vi "KE6221 -- Set Arb Wave Params.vi"(0 "Resource In":refnum<visa-resource-name>, 1 "Check For SCPI Errors? (T)":bool=TRUE, 5 "Arb Location":T1, 7 "Arb Wave Params In":T2={"Frequency (Hz)"=1000.0, "Amplitude (A)"=0.001, "Offset (A)"=0.0, "Ranging Mode"=enum."Best", "Fixed Range"=enum."2mA", "Playback Mode"=enum."Time", "Time (s)"=1.0, "Num Cycles"=1.0, "Phase\nMarker?"=FALSE, "Phase Marker (deg)"=180.0, "Trig Link Line"=enum."1", "Arb Waveform Points"=[], "Num Arb Points"=0} {"Arb Waveform Points" min=-1.0 max=1.0 format="%.3f"; "Offset (A)" min=-0.105 max=0.105 format="%.4p"; "Num Cycles" min=0.001 max=99999999900.0 format="%.3p"; "Time (s)" min=1e-07 max=999999.999 format="%.3p"; "Phase Marker (deg)" min=0.0 max=360.0 format="%.3f"; "Amplitude (A)" min=2e-12 max=0.105 format="%.3p"; "Frequency (Hz)" min=0.001 max=100000.0 format="%.3p"}, 11 "error in (no error)":errorcluster, 12 "Read Back Set Values? (T)":bool=TRUE, 13 "Timeout (10000 ms)":u32=10000) -> (4 "Resource Out (dupl)":refnum<visa-resource-name>, 8 "Arb Wave Params Out":T2={"Frequency (Hz)"=1000.0, "Amplitude (A)"=0.001, "Offset (A)"=0.0, "Ranging Mode"=enum."Best", "Fixed Range"=enum."2mA", "Playback Mode"=enum."Time", "Time (s)"=1.0, "Num Cycles"=1.0, "Phase\nMarker?"=FALSE, "Phase Marker (deg)"=180.0, "Trig Link Line"=enum."1", "Arb Waveform Points"=[], "Num Arb Points"=0} {"Arb Waveform Points" min=-1.0 max=1.0 format="%.3f"; "Offset (A)" min=-0.105 max=0.105 format="%.4p"; "Num Cycles" min=0.001 max=99999999900.0 format="%.3p"; "Time (s)" min=1e-07 max=999999.999 format="%.3p"; "Phase Marker (deg)" min=0.0 max=360.0 format="%.3f"; "Amplitude (A)" min=2e-12 max=0.105 format="%.3p"; "Frequency (Hz)" min=0.001 max=100000.0 format="%.3p"}, 15 "error out":errorcluster)   [LabVIEW 2019, in "Keithley 622x.lvlib"]
doc: "Sets the parameters for an arbitray ('Arb') wave. The user must specify the memory location he wants to write the waveform to, and if it's anything other tha '0 (Volatile)', the waveform will be automatically copied to the non-voltage memory location specified. Note that this VI can only be used with the 6221, since the 6220 doesn't support this feature."
uses:
  Keithley 622x.lvlib
  Typedefs/KE6221 -- Wave Arb Wave Params.ctl
  Low Level/Typedefs/KE6221 -- Wave Frequency.ctl
  Low Level/Typedefs/KE6221 -- Wave Amplitude.ctl
  Source/Typedefs/KE622x -- Current Level.ctl
  Low Level/Typedefs/KE6221 -- Wave Ranging Mode.ctl
  Source/Typedefs/KE622x -- Current Ranges.ctl
  Low Level/Typedefs/KE6221 -- Wave Playback Mode.ctl
  Low Level/Typedefs/KE6221 -- Wave Playback Time.ctl
  Low Level/Typedefs/KE6221 -- Wave Playback Num Cycles.ctl
  Low Level/Typedefs/KE6221 -- Wave Phase Marker.ctl
  Trigger/Low Level/Typedefs/KE622x -- Trig Link Line.ctl
  Low Level/Typedefs/KE6221 -- Wave Arb Point.ctl
  Low Level/Typedefs/KE6221 -- Arb Location.ctl
  Low Level/Typedefs/KE6221 -- Wave Type.ctl
  Source/Typedefs/KE622x -- Current Range.ctl
panel:
  # "Note:  \"Arb Waveform Points\" and \"Num Arb Points\" refer to the Arb waveform in volatile memory (a.k.a. 'Location 0'). For the 'set' VI, the points are automatically copied into the specified non-volatile memory location."
  # "Note:  \"Arb Waveform Points\" and \"Num Arb Points\" refer to the Arb waveform in volatile memory (a.k.a. 'Location 0'). For the 'set' VI, the points are automatically copied into the specified non-volatile memory location."
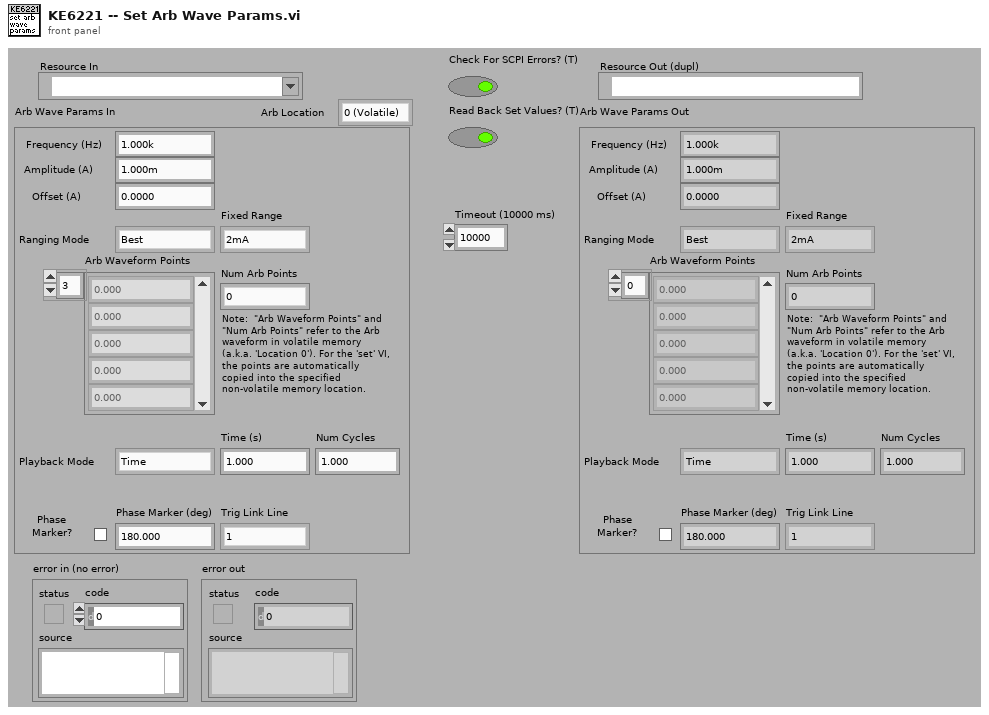
[diagram p1: front panel]
types:
  T1 = typedef "Keithley 622x.lvlib/KE6221 -- Arb Location.ctl" = enum16{"0 (Volatile)", "1 (NVRAM)", "2 (NVRAM)", "3 (NVRAM)", "4 (NVRAM)"}
  T2 = typedef "Keithley 622x.lvlib/KE6221 -- Wave Arb Wave Params.ctl" = cluster{"Frequency (Hz)":T3, "Amplitude (A)":T4, "Offset (A)":T5, "Ranging Mode":T6, "Fixed Range":T7, "Playback Mode":T8, "Time (s)":T9, "Num Cycles":T10, "Phase\nMarker?":bool, "Phase Marker (deg)":T11, "Trig Link Line":T12, "Arb Waveform Points":T13[], "Num Arb Points":u32}
  T3 = typedef "Keithley 622x.lvlib/KE6221 -- Wave Frequency.ctl" = dbl
  T4 = typedef "Keithley 622x.lvlib/KE6221 -- Wave Amplitude.ctl" = dbl
  T5 = typedef "Keithley 622x.lvlib/KE622x -- Current Level.ctl" = dbl
  T6 = typedef "Keithley 622x.lvlib/KE6221 -- Wave Ranging Mode.ctl" = enum16{"Best", "Fixed"}
  T7 = typedef "Keithley 622x.lvlib/KE622x -- Current Ranges.ctl" = enum16{"2nA", "20nA", "200nA", "2uA", "20uA", "200uA", "2mA", "20mA", "100mA"}
  T8 = typedef "Keithley 622x.lvlib/KE6221 -- Wave Playback Mode.ctl" = enum16{"Time", "Num Cycles"}
  T9 = typedef "Keithley 622x.lvlib/KE6221 -- Wave Playback Time.ctl" = dbl
  T10 = typedef "Keithley 622x.lvlib/KE6221 -- Wave Playback Num Cycles.ctl" = dbl
  T11 = typedef "Keithley 622x.lvlib/KE6221 -- Wave Phase Marker.ctl" = dbl
  T12 = typedef "Keithley 622x.lvlib/KE622x -- Trig Link Line.ctl" = enum16{"1", "2", "3", "4", "5", "6"}
  T13 = typedef "Keithley 622x.lvlib/KE6221 -- Wave Arb Point.ctl" = dbl
  T14 = typedef "Keithley 622x.lvlib/KE6221 -- Wave Type.ctl" = enum16{"Sinusoid", "Square", "Ramp", "Arbitrary 0", "Arbitrary 1", "Arbitrary 2", "Arbitrary 3", "Arbitrary 4"}
  T15 = typedef "Keithley 622x.lvlib/KE622x -- Current Range.ctl" = cluster{"Auto Range?":bool, "Man / Selected\nRange":T7}
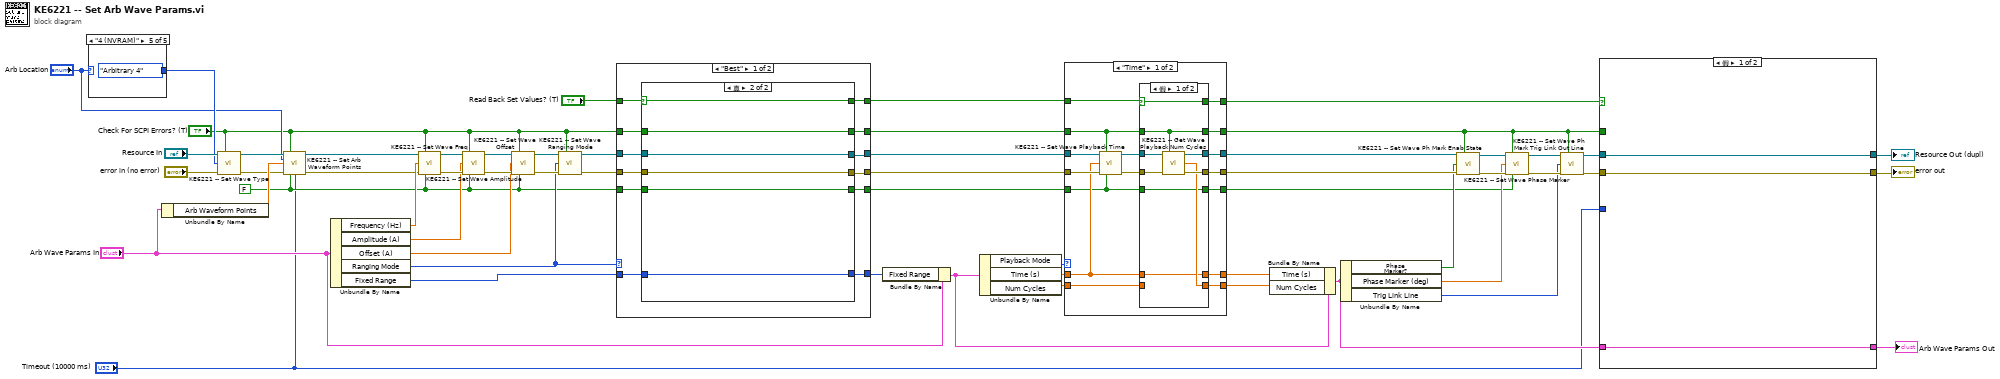
[diagram p0: block diagram]
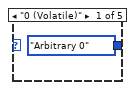
[diagram p2: hidden frame]
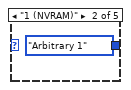
[diagram p3: hidden frame]
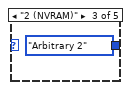
[diagram p4: hidden frame]
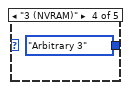
[diagram p5: hidden frame]
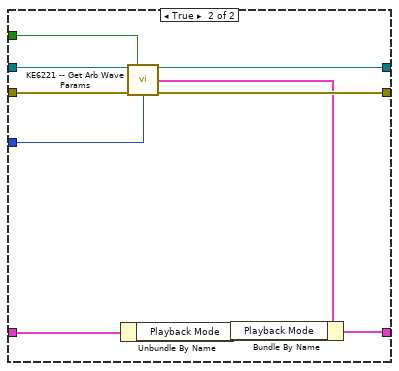
[diagram p6: hidden frame]
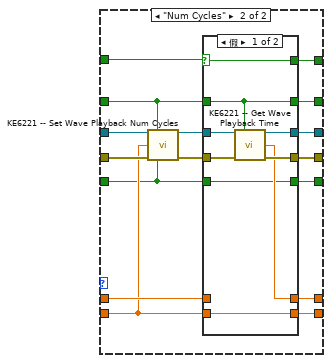
[diagram p8: hidden frame]
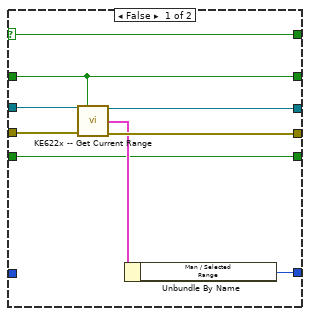
[diagram p10: hidden frame]
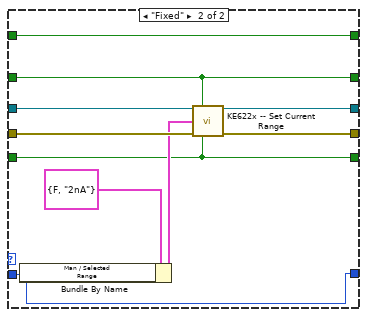
[diagram p11: hidden frame]
diagram:
  w4 = FALSE
  n1 = case shown="\"4 (NVRAM)\"" "Arb Location" {
    tunnel: [KE6221_--_Wave_Type."Arbitrary 0" ("Wave Type") KE6221_--_Wave_Type."Arbitrary 1" ("Wave Type") KE6221_--_Wave_Type."Arbitrary 2" ("Wave Type") KE6221_--_Wave_Type."Arbitrary 3" ("Wave Type") KE6221_--_Wave_Type."Arbitrary 4" ("Wave Type")] -> w14
    frame "0 (Volatile)" {
    }
    frame "1 (NVRAM)" {
    }
    frame "2 (NVRAM)" {
    }
    frame "3 (NVRAM)" {
    }
    frame "4 (NVRAM)" {
    }
  }
  n2 = Unbundle By Name("Arb Wave Params In") -> ("Arb Waveform Points"=w13:T13[])
  n3 = call "KE6221 -- Set Wave Type.vi"("Resource In"="Resource In", "Check For SCPI Errors? (T)"="Check For SCPI Errors? (T)", "Wave Type"=w14, "error in (no error)"="error in (no error)") -> ("Resource Out (dupl)"=w11:refnum<visa-resource-name>, "error out"=w12:errorcluster)  [unwired: 10 in]
  n4 = call "KE6221 -- Set Arb Waveform Points.vi"("Resource In"=w11, "Check For SCPI Errors? (T)"="Check For SCPI Errors? (T)", "Arb Location"="Arb Location", "Arb Waveform Points In"=w13, "error in (no error)"=w12, "Read Back Set Values? (T)"=w4, "Timeout (10 s)"="Timeout (10000 ms)") -> ("Resource Out (dupl)"=w7:refnum<visa-resource-name>, "error out"=w8:errorcluster)  [unwired: 5 in, 2 out]
  n5 = Unbundle By Name("Arb Wave Params In") -> ("Frequency (Hz)"=w45:T3, "Amplitude (A)"=w44:T4, "Offset (A)"=w43:T5, "Ranging Mode"=w42:T6, "Fixed Range"=w41:T7)
  n6 = call "KE6221 -- Set Wave Freq.vi"("Resource In"=w7, "Check For SCPI Errors? (T)"="Check For SCPI Errors? (T)", "Wave Frequency In (Hz)"=w45, "error in (no error)"=w8, "Read Back Set Value? (T)"=w4) -> ("Resource Out (dupl)"=w57:refnum<visa-resource-name>, "error out"=w56:errorcluster)  [unwired: 8 in, 1 out]
  n7 = call "KE6221 -- Set Wave Amplitude.vi"("Resource In"=w57, "Check For SCPI Errors? (T)"="Check For SCPI Errors? (T)", "Wave Amplitude In"=w44, "error in (no error)"=w56, "Read Back Set Value? (T)"=w4) -> ("Resource Out (dupl)"=w53:refnum<visa-resource-name>, "error out"=w52:errorcluster)  [unwired: 8 in, 1 out]
  n8 = call "KE6221 -- Set Wave Offset.vi"("Resource In"=w53, "Check For SCPI Errors? (T)"="Check For SCPI Errors? (T)", "Wave Offset In (A)"=w43, "error in (no error)"=w52, "Read Back Set Value? (T)"=w4) -> ("Resource Out (dupl)"=w51:refnum<visa-resource-name>, "error out"=w50:errorcluster)  [unwired: 8 in, 1 out]
  n9 = call "KE6221 -- Set Wave Ranging Mode.vi"("Resource In"=w51, "Check For SCPI Errors? (T)"="Check For SCPI Errors? (T)", "Ranging Mode"=w42, "error in (no error)"=w50) -> ("Resource Out (dupl)"=w55:refnum<visa-resource-name>, "error out"=w54:errorcluster)  [unwired: 10 in]
  n10 = case shown="\"Best\"" w42 {
    tunnel: w55 -> [w73 w99]
    tunnel: w54 -> [w72 w98]
    tunnel: [w69 w97] -> w38
    tunnel: [w70 w96] -> w35
    tunnel: "Check For SCPI Errors? (T)" -> [w71 w92]
    tunnel: w41 -> [w66 w91]
    tunnel: "Read Back Set Values? (T)" -> [w74 w93]
    tunnel: [w68 w92] -> w34
    tunnel: [w67 w93] -> w33
    tunnel: [w65 w91] -> w32
    tunnel: w4 -> [w64 w90]
    tunnel: [w63 w90] -> w23
    frame "Best" {
      n11 = case shown="真" w74 {
        selector: w74 -> [w78 w89]
        tunnel: w73 -> [w83 w87]
        tunnel: w72 -> [w82 w86]
        tunnel: w71 -> [w79 w88]
        tunnel: [w81 w86] -> w70
        tunnel: [w80 w87] -> w69
        tunnel: [w79 w88] -> w68
        tunnel: [w78 w89] -> w67
        tunnel: w66 -> [_ w85]
        tunnel: [w76 w85] -> w65
        tunnel: w64 -> [w75 w84]
        tunnel: [w75 w84] -> w63
        frame False {
          n12 = call "KE622x -- Get Current Range.vi"("Resource In"=w83, "Check For SCPI Errors? (T)"=w79, "error in (no error)"=w82) -> ("Resource Out (dupl)"=w80:refnum<visa-resource-name>, "Current Range"=w77:T15, "error out"=w81:errorcluster)  [unwired: 10 in]
          n13 = Unbundle By Name(w77) -> ("Man / Selected\nRange"=w76:T7)
        }
        frame True {
        }
      }
    }
    frame "Fixed" {
      n14 = Bundle By Name(cluster=T15 {"Auto Range?"=FALSE, "Man / Selected\nRange"=enum."2nA"} ("Current Range In"), "Man / Selected\nRange"=w91) -> (w94:T15)
      n15 = call "KE622x -- Set Current Range.vi"("Resource In"=w99, "Check For SCPI Errors? (T)"=w92, "Current Range In"=w94, "error in (no error)"=w98, "Read Back Set Values? (T)"=w90) -> ("Resource Out (dupl)"=w97:refnum<visa-resource-name>, "error out"=w96:errorcluster)  [unwired: 8 in, 1 out]
    }
  }
  n16 = Bundle By Name(cluster="Arb Wave Params In", "Fixed Range"=w32) -> (w31:T2)
  n17 = Unbundle By Name(w31) -> ("Playback Mode"=w39:T8, "Time (s)"=w37:T9, "Num Cycles"=w36:T10)
  n18 = case shown="\"Time\"" w39 {
    tunnel: w38 -> [w115 w147]
    tunnel: w37 -> [w104 w138]
    tunnel: w36 -> [w106 w136]
    tunnel: w35 -> [w114 w146]
    tunnel: w34 -> [w110 w142]
    tunnel: w33 -> [w113 w145]
    tunnel: [w105 w135] -> w29
    tunnel: [w109 w141] -> w18
    tunnel: [w108 w140] -> w28
    tunnel: [w107 w139] -> w27
    tunnel: [w103 w137] -> w30
    tunnel: w23 -> [w102 w134]
    tunnel: [w101 w133] -> w22
    tunnel: [w100 w132] -> w21
    frame "Time" {
      n19 = call "KE6221 -- Set Wave Playback Time.vi"("Resource In"=w115, "Check For SCPI Errors? (T)"=w110, "Playback Time (s) In"=w104, "error in (no error)"=w114, "Read Back Set Value? (T)"=w102) -> ("Resource Out (dupl)"=w112:refnum<visa-resource-name>, "error out"=w111:errorcluster)  [unwired: 8 in, 1 out]
      n20 = case shown="假" w113 {
        selector: w113 -> [w116 w125]
        tunnel: w112 -> [w124 w129]
        tunnel: w111 -> [w123 w130]
        tunnel: w110 -> [w122 w131]
        tunnel: [w122 w131] -> w109
        tunnel: [w121 w130] -> w107
        tunnel: [w120 w129] -> w108
        tunnel: w106 -> [_ w128]
        tunnel: [w119 w128] -> w105
        tunnel: w104 -> [w118 w127]
        tunnel: [w118 w127] -> w103
        tunnel: w102 -> [w117 w126]
        tunnel: [w117 w126] -> w101
        tunnel: [w116 w125] -> w100
        frame False {
          n21 = call "KE6221 -- Get Wave Playback Num Cycles.vi"("Resource In"=w124, "Check For SCPI Errors? (T)"=w122, "error in (no error)"=w123) -> ("Resource Out (dupl)"=w120:refnum<visa-resource-name>, "Num Cycles"=w119:T10, "error out"=w121:errorcluster)  [unwired: 10 in]
        }
        frame True {
        }
      }
    }
    frame "Num Cycles" {
      n22 = call "KE6221 -- Set Wave Playback Num Cycles.vi"("Resource In"=w147, "Check For SCPI Errors? (T)"=w142, "Num Cycles In"=w136, "error in (no error)"=w146, "Read Back Set Value? (T)"=w134) -> ("Resource Out (dupl)"=w144:refnum<visa-resource-name>, "error out"=w143:errorcluster)  [unwired: 8 in, 1 out]
      n23 = case shown="假" w145 {
        selector: w145 -> [w148 w157]
        tunnel: w144 -> [w156 w161]
        tunnel: w143 -> [w155 w162]
        tunnel: w142 -> [w154 w163]
        tunnel: [w154 w163] -> w141
        tunnel: [w153 w162] -> w139
        tunnel: [w152 w161] -> w140
        tunnel: w138 -> [_ w160]
        tunnel: [w151 w160] -> w137
        tunnel: w136 -> [w150 w159]
        tunnel: [w150 w159] -> w135
        tunnel: w134 -> [w149 w158]
        tunnel: [w149 w158] -> w133
        tunnel: [w148 w157] -> w132
        frame False {
          n24 = call "KE6221 -- Get Wave Playback Time.vi"("Resource In"=w156, "Check For SCPI Errors? (T)"=w154, "error in (no error)"=w155) -> ("Resource Out (dupl)"=w152:refnum<visa-resource-name>, "Playback Time (s)"=w151:T9, "error out"=w153:errorcluster)  [unwired: 10 in]
        }
        frame True {
        }
      }
    }
  }
  n25 = Bundle By Name(cluster=w31, "Time (s)"=w30, "Num Cycles"=w29) -> (w17:T2)
  n26 = Unbundle By Name(w17) -> ("Phase\nMarker?"=w26:bool, "Phase Marker (deg)"=w25:T11, "Trig Link Line"=w24:T12)
  n27 = call "KE6221 -- Set Wave Ph Mark Enab State.vi"("Resource In"=w28, "Check For SCPI Errors? (T)"=w18, "Phase Marker Enabled?"=w26, "error in (no error)"=w27) -> ("Resource Out (dupl)"=w49:refnum<visa-resource-name>, "error out"=w48:errorcluster)  [unwired: 10 in]
  n28 = call "KE6221 -- Set Wave Phase Marker.vi"("Resource In"=w49, "Check For SCPI Errors? (T)"=w18, "Phase Marker In (deg)"=w25, "error in (no error)"=w48, "Read Back Set Value? (T)"=w22) -> ("Resource Out (dupl)"=w47:refnum<visa-resource-name>, "error out"=w46:errorcluster)  [unwired: 8 in, 1 out]
  n29 = call "KE6221 -- Set Wave Ph Mark Trig Link Out Line.vi"("Resource In"=w47, "Check For SCPI Errors? (T)"=w18, "Trig Link Out Line"=w24, "error in (no error)"=w46) -> ("Resource Out (dupl)"=w20:refnum<visa-resource-name>, "error out"=w19:errorcluster)  [unwired: 10 in]
  n30 = case shown="假" w21 {
    tunnel: w20 -> [w165 w176]
    tunnel: w19 -> [w164 w175]
    tunnel: w18 -> [_ w174]
    tunnel: [w165 w173] -> w2
    tunnel: [w164 w172] -> w1
    tunnel: w17 -> [w166 w171]
    tunnel: [w166 w168] -> w5
    tunnel: "Timeout (10000 ms)" -> [_ w167]
    frame False {
    }
    frame True {
      n31 = Unbundle By Name(w171) -> ("Playback Mode"=w169:T8)
      n32 = call "KE6221 -- Get Arb Wave Params.vi"("Resource In"=w176, "Check For SCPI Errors? (T)"=w174, "error in (no error)"=w175, "Timeout (10000 ms)"=w167) -> ("Resource Out (dupl)"=w173:refnum<visa-resource-name>, "Arb Wave Params"=w170:T2, "error out"=w172:errorcluster)  [unwired: 9 in]
      n33 = Bundle By Name(cluster=w170, "Playback Mode"=w169) -> (w168:T2)
    }
  }
  "Resource Out (dupl)" <- w2
  "error out" <- w1
  "Arb Wave Params Out" <- w5
